vi "ScratchPad.vi"() -> ()   [LabVIEW 2020, in "Parallel Block.lvlib"]
uses:
  Parallel Block.lvlib
  Type Descriptor/Type Descriptor.lvclass
  Value Type.ctl
  f8d29441-1da7-4d0b-a8ee-9ca22e0245ab.vi
  f8d29441-1da7-4d0b-a8ee-9ca22e0245ab.vi/3bed3f69-881b-4068-86a2-eab8f40400a4.vi
  Type Descriptor/Set Type Descriptor.vi
panel:
  out "String":string
  out "Value Type":T1
  out "Default":variant=variant(cluster{"x0":dbl, "dx":dbl, "y":cdb[]} {"x0"=0.0, "dx"=0.0, "y"=[]})
  out "Type Descriptor":refnum<class "Type Descriptor.lvclass">
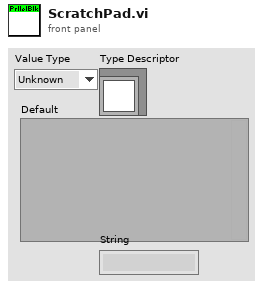
[diagram p1: front panel]
types:
  T1 = typedef "Parallel Block.lvlib/Value Type.ctl" = enum16{"Unknown", "Bool", "U8", "U16", "U32", "U64", "I8", "I16", "I32", "I64", "SGL", "DBL", "CSG", "CDB", "CDBWFM", "String"}
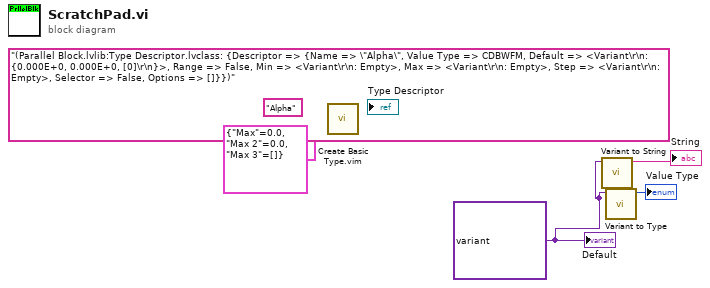
[diagram p0: block diagram]
diagram:
  (unwired) "(Parallel Block.lvlib:Type Descriptor.lvclass: {Descriptor => {Name => \"Alpha\", Value Type => CDBWFM, Default => <Variant\r\n: {0.000E+0, 0.000E+0, [0]\r\n}>, Range => False, Min => <Variant\r\n: Empty>, Max => <Variant\r\n: Empty>, Step => <Variant\r\n: Empty>, Selector => False, Options => []}})"
  w2 = variant(cluster{"x0":dbl, "dx":dbl, "y":cdb[]} {"x0"=0.0, "dx"=0.0, "y"=[]}) ("Default")
  n1 = call "Create Basic Type.vim"("Type & Default"=cluster{"Max":dbl, "Max 2":dbl, "Max 3":cdb[]} {"Max"=0.0, "Max 2"=0.0, "Max 3"=[]}, "Name"="Alpha") -> ("Type Descriptor"=→"Type Descriptor":refnum<class "Type Descriptor.lvclass">)  [unwired: 9 in]
  n2 = call "Variant to String.vi"("Value"=w2) -> ("String"=→"String":string)  [unwired: 10 in]
  n3 = call "Variant to Type.vi"("Value"=w2) -> ("Value Type"=→"Value Type":T1)  [unwired: 10 in]
  "Default" <- w2
